vi "Connect.vi"(8 "error in (no error)":errorcluster, 10 "Timeout":i32=2000, 11 "ClientBase in":refnum<class "TCP.lvclass">) -> (0 "error out":errorcluster, 3 "ClientBase out":refnum<class "TCP.lvclass">)   [LabVIEW 2020, in "TCP.lvlib" / "TCP.lvclass"]
uses:
  TCP.lvclass
  TCP.lvclass/TCP.ctl
  <vilib>/net/WFCN/NI_WFCN.lvlib
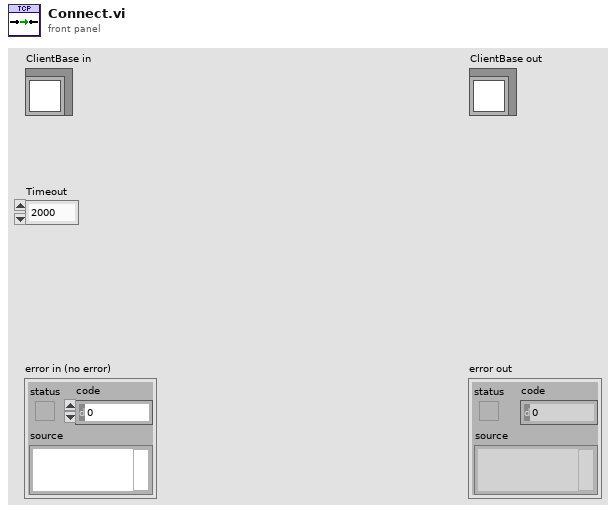
[diagram p1: front panel]
types:
  T1 = typedef "NI_WFCN.lvlib/Network Status.ctl" = enum16{"Indeterminate", "Configured", "Unconfigured"}
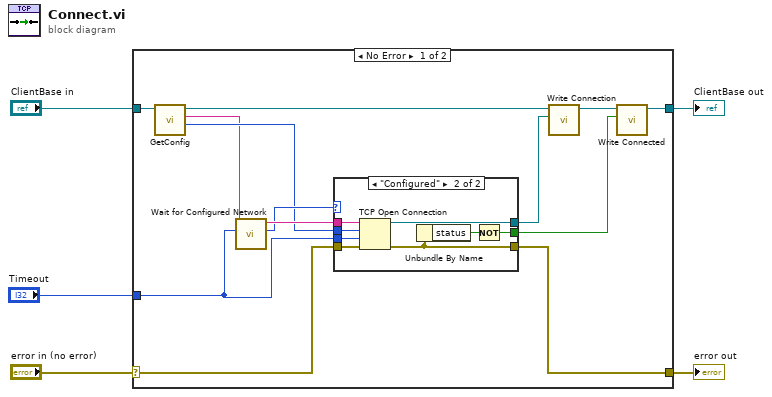
[diagram p0: block diagram]
diagram:
  n1 = case shown="No Error" "error in (no error)" {
    selector: "error in (no error)" -> [w18 w29]
    tunnel: [w17 w29] -> w4
    tunnel: [w7 w28] -> w2
    tunnel: "ClientBase in" -> [w12 w28]
    tunnel: "Timeout" -> [w6 _]
    frame No Error {
      n2 = call "GetConfig.vi"("ClientBase in"=w12) -> ("Port"=w14:u16, "Address"=w13:string, "ClientBase out"=w8:refnum<class "TCP.lvclass">)  [unwired: 6 in, 2 out]
      n3 = call <vilib>:"Wait for Configured Network.vi"("timeout in ms"=w6, "hostname or URL in"=w13) -> ("network status for remote host"=w15:T1, "hostname or URL out"=w16:string)  [unwired: 8 in]
      n4 = case shown="\"Configured\"" w15 {
        tunnel: w14 -> [_ w27]
        tunnel: w18 -> [w19 w26]
        tunnel: [w19 w22] -> w17
        tunnel: [_ w25] -> w10
        tunnel: w6 -> [_ w24]
        tunnel: w16 -> [_ w23]
        tunnel: [_ w20] -> w11
        frame "Indeterminate", Default {
        }
        frame "Configured" {
          n5 = TCP Open Connection(address=w23, remote port or service name=w27, timeout ms (60000)=w24, error in (no error)=w26) -> (connection ID=w25:refnum<k5>, error out=w22:errorcluster)  [unwired: 1 in]
          n6 = Unbundle By Name(w22) -> ("status"=w21:bool)
          n7 = Not(x=w21) -> (.not. x?=w20:bool)
        }
      }
      n8 = call "Write Connection.vi"("Connection ID"=w10, "ClientBase in"=w8) -> ("ClientBase out"=w9:refnum<class "TCP.lvclass">)  [unwired: 8 in, 1 out]
      n9 = call "Write Connected.vi"("Connected"=w11, "ClientBase in"=w9) -> ("ClientBase out"=w7:refnum<class "TCP.lvclass">)  [unwired: 8 in, 1 out]
    }
    frame Error {
    }
  }
  "error out" <- w4
  "ClientBase out" <- w2
